vi "readFromXML.vi"(8 "error in (no error)":errorcluster, 10 "XMLin":string, 11 "FixedTarget in":refnum<class "FixedTarget.lvclass">) -> (0 "error out":errorcluster, 3 "FixedTarget out":refnum<class "FixedTarget.lvclass">)   [LabVIEW 2022 SP3, in "TCSDataDefinitions.lvlib" / "TCSCommand.lvlib" / "TargetConfiguration.lvlib" / "Target.lvlib" / "FixedTarget.lvlib" / "FixedTarget.lvclass"]
uses:
  FixedTarget.lvclass
  <userlib>/Common/UnitsAndXML/FlattenItemWithUnitToXML/FlattenPlaneAngleToXML/PlaneAngleUnit.ctl
  <userlib>/Common/UnitsAndXML/FlattenItemWithUnitToXML/FlattenVelocityToXML/VelocityUnit.ctl
  FixedTarget.lvclass/FixedTarget.ctl
  Target/Target.lvclass
  ProperMotion/ProperMotion.lvclass
  <userlib>/Common/UnitsAndXML/UnitsAndXML.lvlib
  <userlib>/Common/XML/XMLParser/XMLParser.lvclass
panel:
  out "targetName":string
  out "rv_kps":dbl[unit]
  out "parallax":dbl[unit]
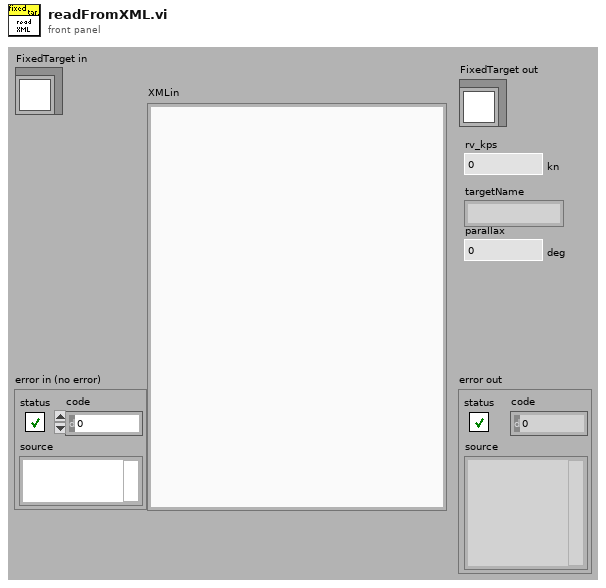
[diagram p1: front panel]
types:
  T1 = typedef "UnitsAndXML.lvlib/VelocityUnit.ctl" = enum16{"m/s", "km/s", "kn"}
  T2 = typedef "UnitsAndXML.lvlib/PlaneAngleUnit.ctl" = enum16{"rad", "deg", "'", "\""}
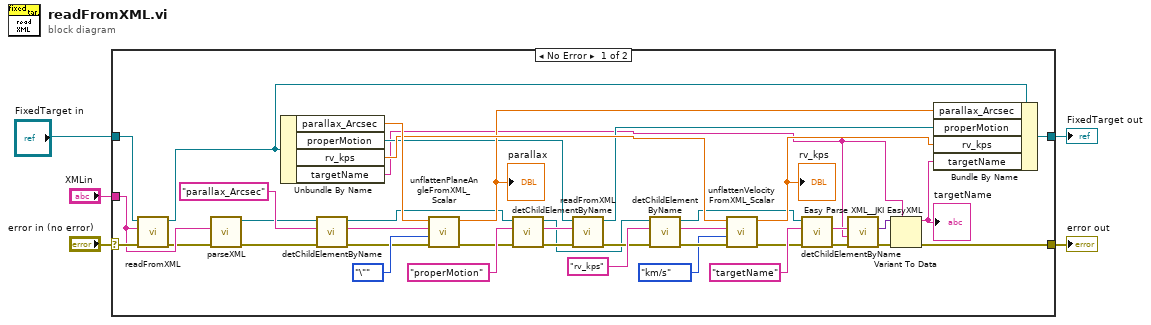
[diagram p0: block diagram]
diagram:
  n1 = case shown="No Error" "error in (no error)" {
    selector: "error in (no error)" -> [w44 w46]
    tunnel: [w12 w46] -> w4
    tunnel: [w36 w45] -> w3
    tunnel: "FixedTarget in" -> [w11 w45]
    tunnel: "XMLin" -> [w43 _]
    frame No Error {
      n2 = call-parent "readFromXML.vi"("error in (no error)"=w44, "XML in"=w43, "Target in"=w11) -> ("error out"=w42:errorcluster, "Target out"=w10:refnum<class "FixedTarget.lvclass">)  [unwired: 7 in]
      n3 = call <userlib>:"parseXML.vi"("error in (no error)"=w42, "XMLString in"=w43) -> ("error out"=w40:errorcluster, "Element out"=w9:refnum<class "XMLParser.lvclass">)  [unwired: 8 in]
      n4 = Unbundle By Name(w10) -> ("parallax_Arcsec"=w35:dbl[unit], "properMotion"=w23:refnum<class "ProperMotion.lvclass">, "rv_kps"=w26:dbl[unit], "targetName"=w14:string)
      n5 = call <userlib>:"detChildElementByName.vi"("error in (no error)"=w40, "childName"="parallax_Arcsec" ("ChildName"), "Element in"=w9) -> ("error out"=w32:errorcluster, "childXML"=w34:string, "Element out"=w8:refnum<class "XMLParser.lvclass">)  [unwired: 5 in, 1 out]
      n6 = call <userlib>:"unflattenPlaneAngleFromXML_Scalar.vi"("error in (no error)"=w32, "planeAngleUnitInXML"=PlaneAngleUnit."\"", "xmlString"=w34, "planeAngleForType"=w35) -> ("error out"=w31:errorcluster, "planeAngle"=w24:dbl[unit])  [unwired: 6 in]
      "parallax" <- w24
      n7 = call <userlib>:"detChildElementByName.vi"("error in (no error)"=w31, "childName"="properMotion" ("ChildName"), "Element in"=w8) -> ("error out"=w20:errorcluster, "childXML"=w22:string, "Element out"=w7:refnum<class "XMLParser.lvclass">)  [unwired: 5 in, 1 out]
      n8 = call-dynamic "readFromXML.vi"("error in (no error)"=w20, "XML in"=w22, "ProperMotion in"=w23) -> ("error out"=w19:errorcluster, "ProperMotion out"=w21:refnum<class "ProperMotion.lvclass">)  [unwired: 7 in]
      n9 = call <userlib>:"detChildElementByName.vi"("error in (no error)"=w19, "childName"="rv_kps" ("ChildName"), "Element in"=w7) -> ("error out"=w30:errorcluster, "childXML"=w27:string, "Element out"=w6:refnum<class "XMLParser.lvclass">)  [unwired: 5 in, 1 out]
      n10 = call <userlib>:"unflattenVelocityFromXML_Scalar.vi"("error in (no error)"=w30, "velocityUnitInXML"=VelocityUnit."km/s", "xmlString"=w27, "velocityForType"=w26) -> ("error out"=w29:errorcluster, "velocity"=w25:dbl[unit])  [unwired: 6 in]
      "rv_kps" <- w25
      n11 = call <userlib>:"detChildElementByName.vi"("error in (no error)"=w29, "childName"="targetName" ("ChildName"), "Element in"=w6) -> ("error out"=w17:errorcluster, "childXML"=w18:string)  [unwired: 5 in, 2 out]
      n12 = call <vilib>:"Easy Parse XML__JKI EasyXML.vi"("error in (no error)"=w17, "LabVIEW Data (Type)"=w14, "XML String"=w18) -> ("error out"=w16:errorcluster, "LabVIEW Data"=w15:variant)  [unwired: 7 in]
      n13 = Variant To Data(error in=w16, type=w14, Variant=w15) -> (data=w13:string, error out=w12:errorcluster)
      "targetName" <- w13
      n14 = Bundle By Name(cluster=w10, "parallax_Arcsec"=w24, "properMotion"=w21, "rv_kps"=w25, "targetName"=w13) -> (w36:refnum<class "FixedTarget.lvclass">)
    }
    frame Error {
    }
  }
  "error out" <- w4
  "FixedTarget out" <- w3
